vi "qSVA.vi"(0 "System no.":i32=1 min=1 max=4 step=1, 2 "Axes to query":string[](array[string]), 3 "All axes?":bool, 4 "Axis identifier?":bool=TRUE, 5 "error in":errorcluster) -> (14 "Commanded PZT voltage":dbl[](array[numeric]) format="%.6f", 19 "error out":errorcluster)   [LabVIEW 2026]
doc: "Returns commanded PZT voltage for queried axes.\n\nE-516, E-710: If All axes= TRUE, then Axis identifier? must be TRUE\n\nC-413, E-517, E-518, E-709, E-712, E-725, E-727, E-753, E-754, E-755, E-761, E-874: If All axes= TRUE, then Axis identifier? can be FALSE. \n\nE-712, E-725, E-727, E-753, E-754, E-761: The response is a dimensionsless value whose range corresponds approximately to the mechanics travel range in µm.\n\nE-816: All axes? = FALSE, only one axis per command allowed."
panel:
  # "Returns commanded PZT voltage for queried axes."
  # "If all axes: use"
  # "Query"
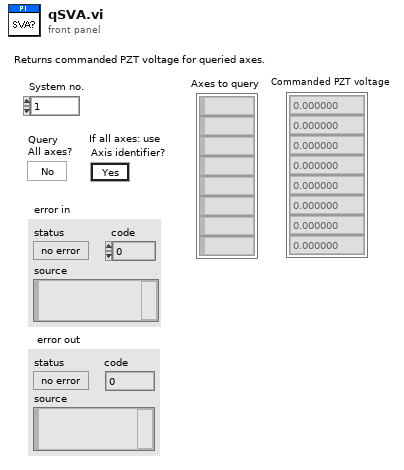
[diagram p1: front panel]
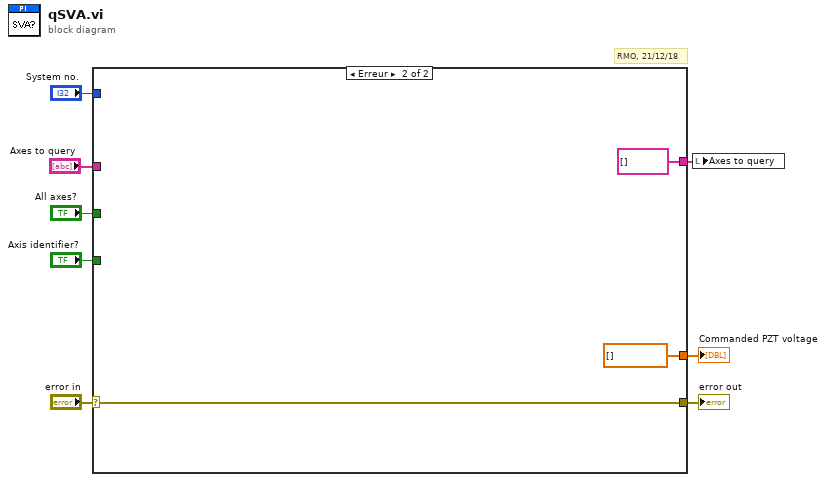
[diagram p0: block diagram]
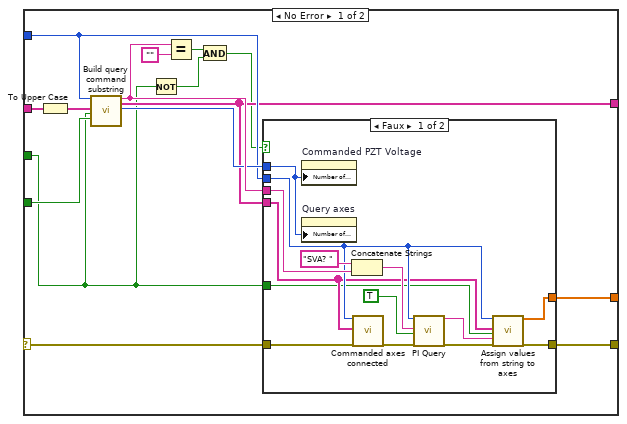
[diagram p2: hidden frame]
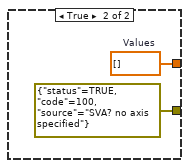
[diagram p3: hidden frame]
diagram:
  # "RMO, 21/12/18"
  n1 = case shown="Erreur" "error in" {
    selector: "error in" -> [w9 w40]
    tunnel: [w23 dbl[] [] ("Values")] -> w8
    tunnel: "Axes to query" -> [w22 _]
    tunnel: [w11 w40] -> w6
    tunnel: "Axis identifier?" -> [w19 _]
    tunnel: "System no." -> [w16 _]
    tunnel: [w15 string[] [] ("Axes to query out")] -> w3
    tunnel: "All axes?" -> [w14 _]
    frame No Error {
      n2 = To Upper Case(1:w22) -> (0:w20:string[])
      n3 = call "Build query command substring.vi"("System no."=w16, "Axes to query in"=w20, "Query\nAll axes?"=w14, "For all axes: use\nAxis identifier?"=w19) -> ("Command substring"=w18:string, "Axes to query out"=w15:string[], "Number of rows"=w17:u32)  [unwired: 2 in, 11 out]
      n4 = Not(x=w14) -> (.not. x?=w12:bool)
      n5 = Equal?(x=w18, y="" ("x")) -> (x = y?=w13:bool)
      n6 = And(x=w13, y=w12) -> (x .and. y?=w10:bool)
      n7 = case shown="Faux" w10 {
        tunnel: [w34 w38] -> w23
        tunnel: w9 -> [w33 _]
        tunnel: w18 -> [w32 _]
        tunnel: w17 -> [w31 _]
        tunnel: w16 -> [w30 _]
        tunnel: w15 -> [w29 _]
        tunnel: w14 -> [w28 _]
        tunnel: [w26 errorcluster {"status"=TRUE, "code"=100, "source"="SVA? no axis specified"} ("error out")] -> w11
        frame False {
          n8 = property on="Commanded PZT Voltage" class="Tabl (strict)"("Number of Rows"=w31) -> ()  [unwired: 2 in, 2 out]
          n9 = property on="Query axes" class="Tabl (strict)"("Number of Rows"=w31) -> ()  [unwired: 2 in, 2 out]
          n10 = Concatenate Strings("SVA? ", w32) -> (w35:string)
          n11 = call "Commanded axes connected.vi"("System no."=w30, "Commanded axes"=w29, "error in"=w33) -> ("error out"=w27:errorcluster)  [unwired: 1 in, 15 out]
          n12 = call "PI Query.vi"("System no."=w30, "String to send"=w35, "Attach termination char.?"=TRUE ("Attach Linefeed?"), "error in"=w27) -> ("String read"=w24:string, "error out"=w25:errorcluster)  [unwired: 3 in, 11 out]
          n13 = call "Assign values from string to axes.vi"("System no."=w30, "Queried axes"=w29, "All axes queried?"=w28, "Input String"=w24, "error in"=w25) -> ("Values"=w34:dbl[], "error out"=w26:errorcluster)  [unwired: 4 in, 9 out]
        }
        frame True {
          w38 = dbl[] []  # Values
        }
      }
    }
    frame Error {
    }
  }
  "error out" <- w6
  "Commanded PZT voltage" <- w8
  n14 = local write "Axes to query"(w3) -> ()
